vi "Agitator Settings Dialog.vi"(8 "error in (no error)":errorcluster, 10 "Message Queues":T7, 11 "Agitator Module State Cluster In":T1={"State"=enum."Idle", "Start Time"=timestamp(0 s since 1904-01-01), "Current Time"=timestamp(0 s since 1904-01-01), "Agitator Module Config"={"GUID"="", "Drop Coords"={"Horizontal"=0, "Vertical"=0}, "Process Name"="", "User name"="", "Queue Name"="", "Settings"={"Cycle Period"=500.0, "Agitator Type"="", "Setpoint (µm)"=0.0, "IKA EUROSTAR Settings"={"VISA resource name"="", "Simulated?"=FALSE}}, "Load Count"=0}, "Output Error"=FALSE, "Log Started"=FALSE, "First Iteration"=FALSE, "Data"={"Agitator rpm Value"=0.0}, "Agitator On?"=enum."Off"}) -> (0 "error out":errorcluster, 1 "Cancelled?":bool=TRUE, 2 "UI Refresh Needed?":bool, 3 "Agitator Module State Cluster Out":T1={"State"=enum."Idle", "Start Time"=timestamp(0 s since 1904-01-01), "Current Time"=timestamp(0 s since 1904-01-01), "Agitator Module Config"={"GUID"="", "Drop Coords"={"Horizontal"=0, "Vertical"=0}, "Process Name"="", "User name"="", "Queue Name"="", "Settings"={"Cycle Period"=500.0, "Agitator Type"="", "Setpoint (µm)"=0.0, "IKA EUROSTAR Settings"={"VISA resource name"="", "Simulated?"=FALSE}}, "Load Count"=0}, "Output Error"=FALSE, "Log Started"=FALSE, "First Iteration"=FALSE, "Data"={"Agitator rpm Value"=0.0}, "Agitator On?"=enum."Off"})   [LabVIEW 2018, in "Agitator Module.lvlib"]
doc: "Dialog for selecting user specified settings."
uses:
  Agitator Module.lvlib
  Feed Module/Controls/Agitator Module Settings Cluster and Start Stop.ctl
  Feed Module/Controls/Agitator Module Settings Cluster.ctl
  IKA EUROSTAR/IKA EUROSTAR Settings.ctl
  Agitator Message Queues.ctl
  support/Message Queue/Message Cluster.ctl
  Feed Module/Controls/Agitator Module State Cluster.ctl
  Pump Module Folder/Measure Instrument/State Enum.ctl
  Feed Module/Controls/Agitator Module Config Cluster.ctl
  <vilib>/Utility/miscctls.llb/LVPoint32TypeDef.ctl
  support/Message Queue/Enqueue Message (Single).vi
  <vilib>/Utility/xml.llb/Write to XML File(string).vi
  Settings/Settings.lvlib
  Measure Instrument/Agitator Module Engine.lvlib
  support/Support Library.lvlib
  support/Message Queue/Message Queue.lvlib
  Pump Module Folder/Measure Instrument/Pump Module Engine.lvlib
  IKA EUROSTAR/IKA EUROSTAR.lvlib
panel:
  in  "Configuration + Buttons":T8={"Configuration"={"Cycle Period"=500.0, "Agitator Type"="", "Setpoint (µm)"=0.0, "IKA EUROSTAR Settings"={"VISA resource name"="", "Simulated?"=FALSE}}, "Stop"=FALSE, "Start"=FALSE}
  in  "Module Name":string
  in  "Cancel Button":bool
  in  "OK Button":bool
  # "Non visible portion of dialog (needed for connector pane)."
  # "Agitator Settings"
  # "Agitator Settings"
  # "Agitator Settings"
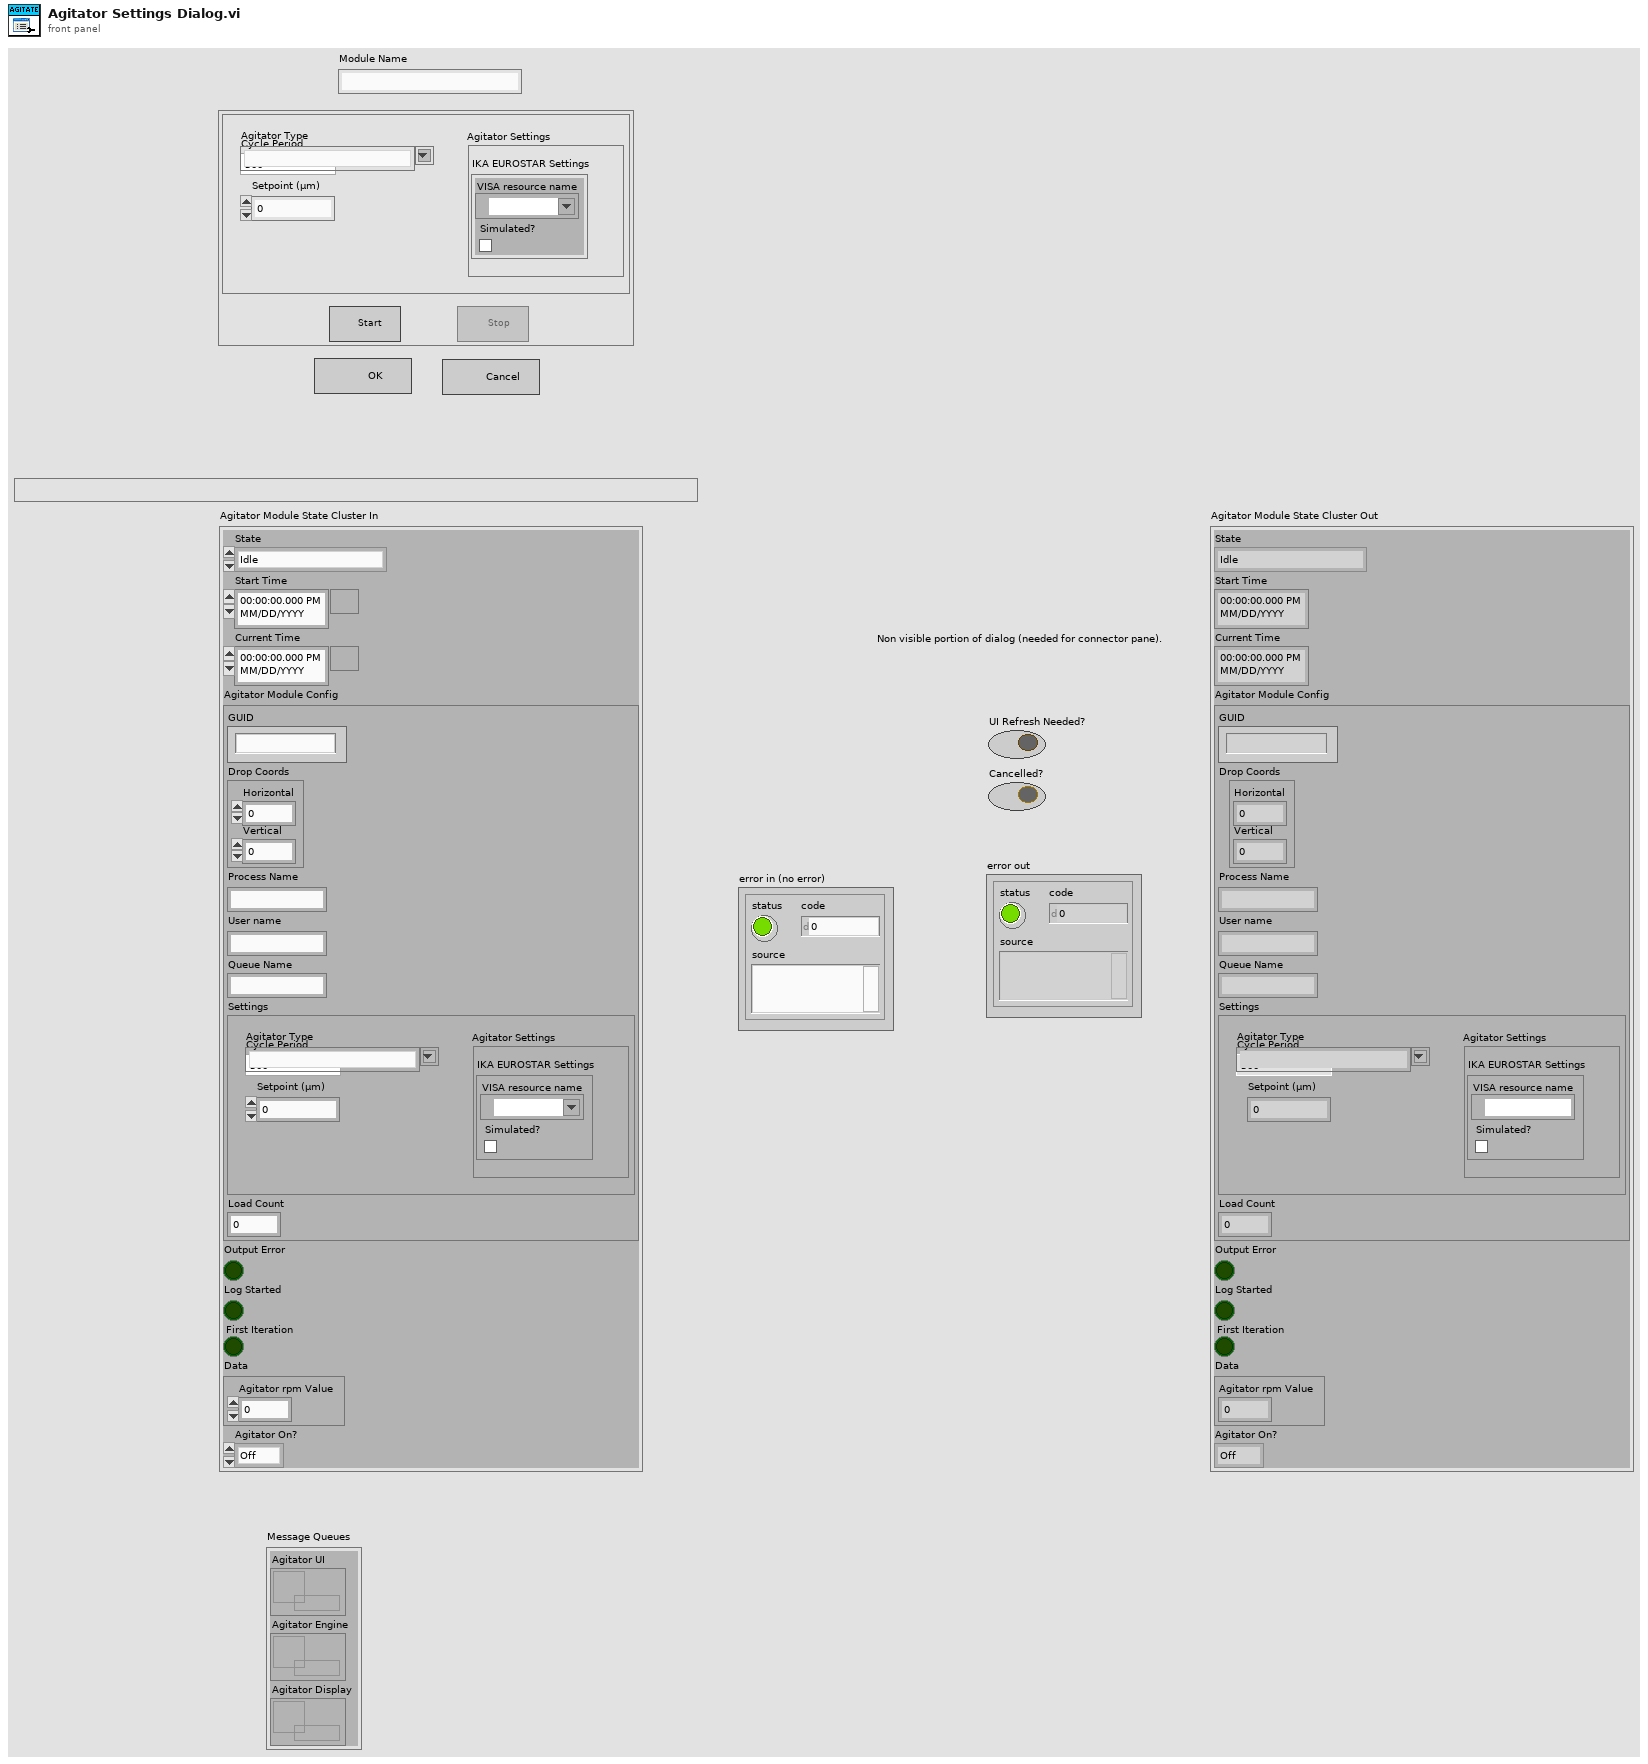
[diagram p1: front panel]
types:
  T1 = typedef "Agitator Module.lvlib/Agitator Module State Cluster.ctl" = cluster{"State":T2, "Start Time":timestamp, "Current Time":timestamp, "Agitator Module Config":T3, "Output Error":bool, "Log Started":bool, "First Iteration":bool, "Data":cluster{"Agitator rpm Value":dbl}, "Agitator On?":enum16{"Off", "On", "Not Initialized", "Over Cutoff"}}
  T2 = typedef "Pump Module.lvlib/Pump Module Engine.lvlib/State Enum.ctl" = enum16{"Measuring", "Idle", "Paused"}
  T3 = typedef "Agitator Module.lvlib/Agitator Module Config Cluster.ctl" = cluster{"GUID":string, "Drop Coords":T4, "Process Name":string, "User name":string, "Queue Name":string, "Settings":T5, "Load Count":i32}
  T4 = typedef "LVPoint32TypeDef.ctl" = cluster{"Horizontal":i32, "Vertical":i32}
  T5 = typedef "Agitator Module.lvlib/Agitator Module Settings Cluster.ctl" = cluster{"Cycle Period":dbl, "Agitator Type":string, "Setpoint (µm)":dbl, "IKA EUROSTAR Settings":T6}
  T6 = typedef "IKA EUROSTAR.lvlib/IKA EUROSTAR Settings.ctl" = cluster{"VISA resource name":refnum<visa-resource-name>, "Simulated?":bool}
  T7 = typedef "Agitator Module.lvlib/Agitator Message Queues.ctl" = cluster{"Agitator UI":refnum<queue>, "Agitator Engine":refnum<queue>, "Agitator Display":refnum<queue>}
  T8 = typedef "Agitator Module.lvlib/Agitator Module Settings Cluster and Start Stop.ctl" = cluster{"Configuration":T5, "Stop":bool, "Start":bool}
  T9 = enum8{"Enabled", "Disabled", "Disabled and Grayed Out"}
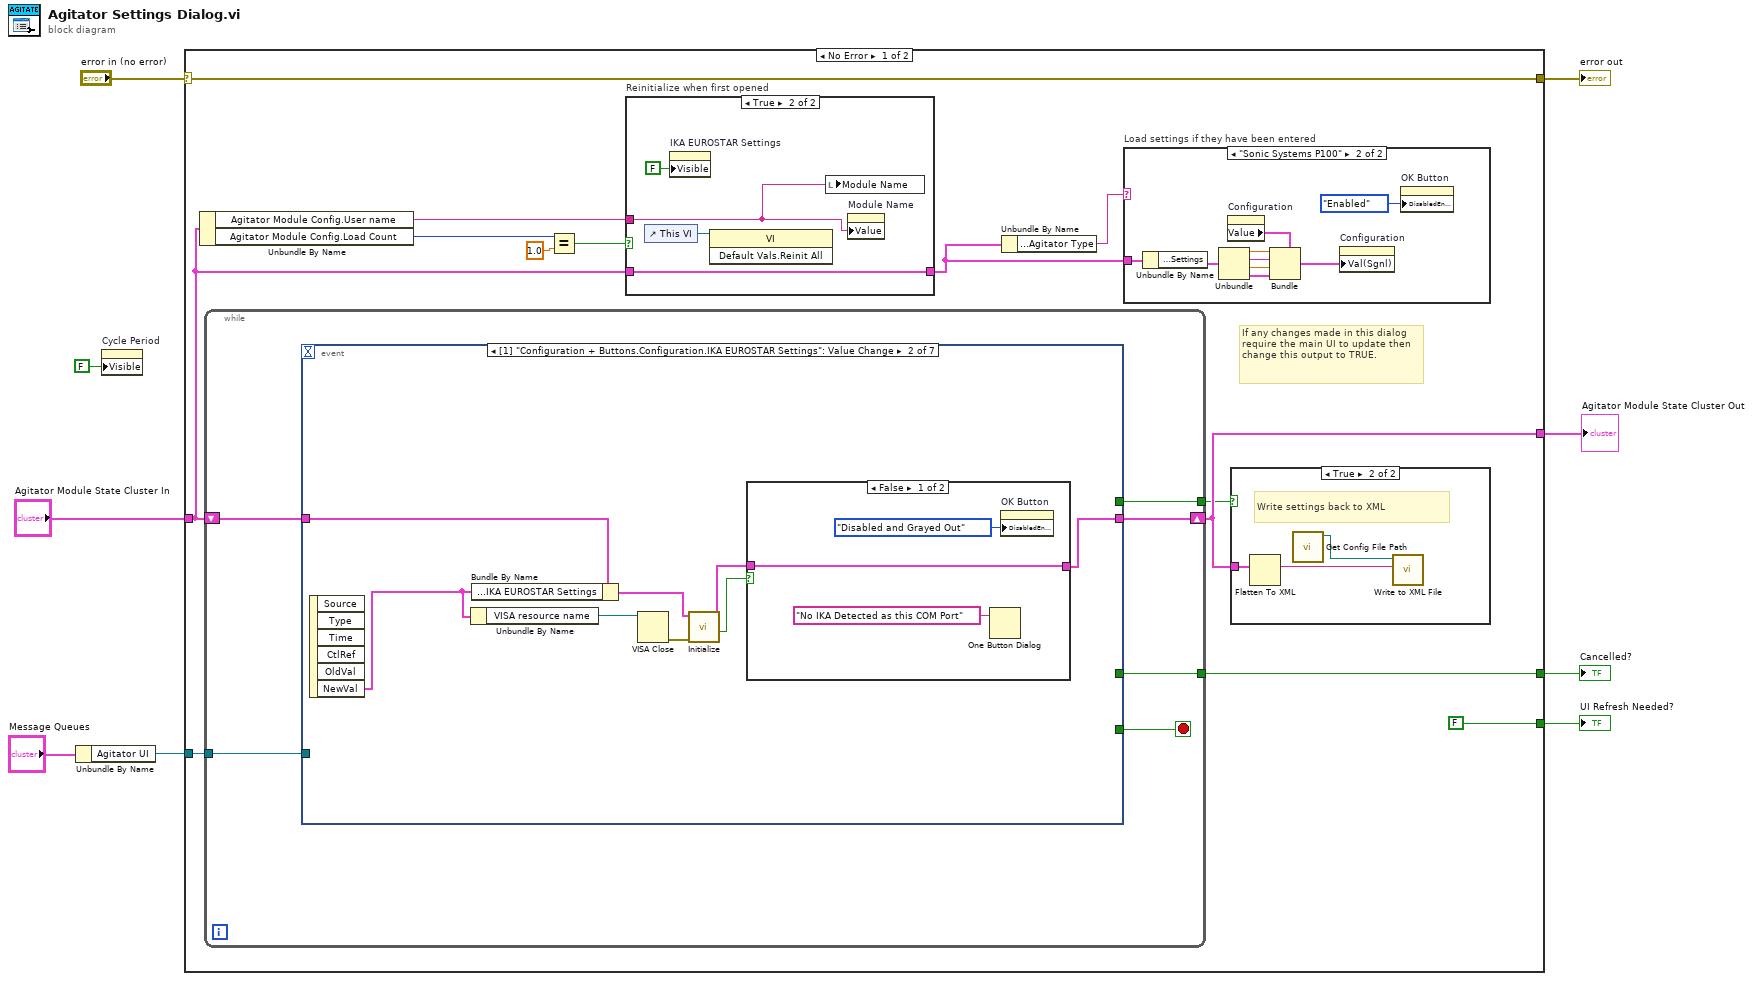
[diagram p0: block diagram]
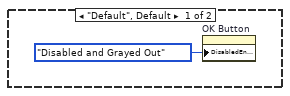
[diagram p2: hidden frame]
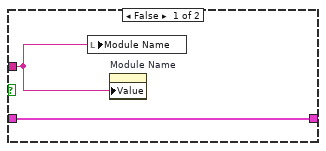
[diagram p3: hidden frame]
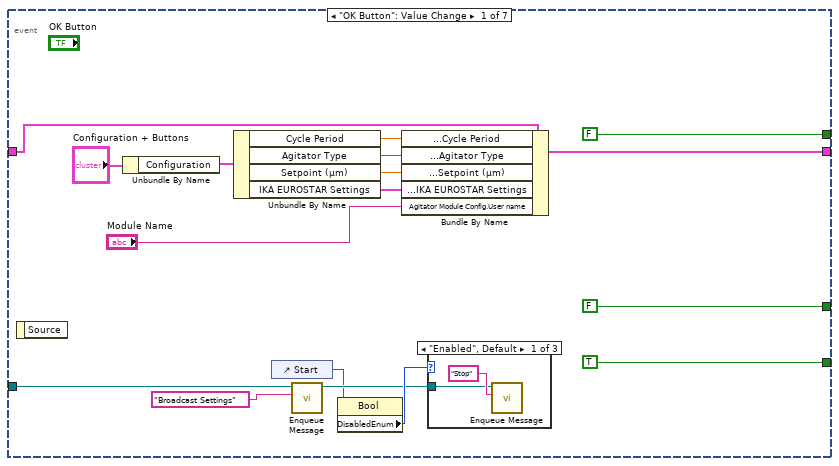
[diagram p4: hidden frame]
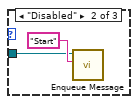
[diagram p5: hidden frame]
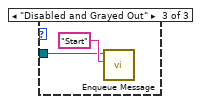
[diagram p6: hidden frame]
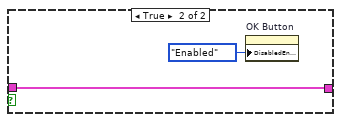
[diagram p7: hidden frame]
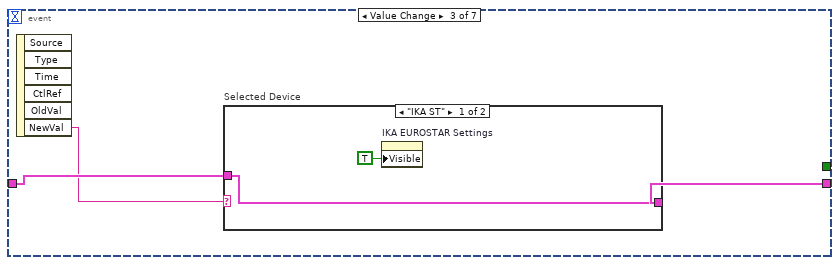
[diagram p8: hidden frame]
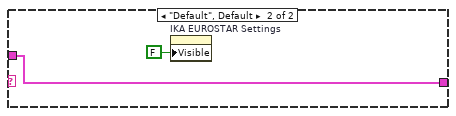
[diagram p9: hidden frame]
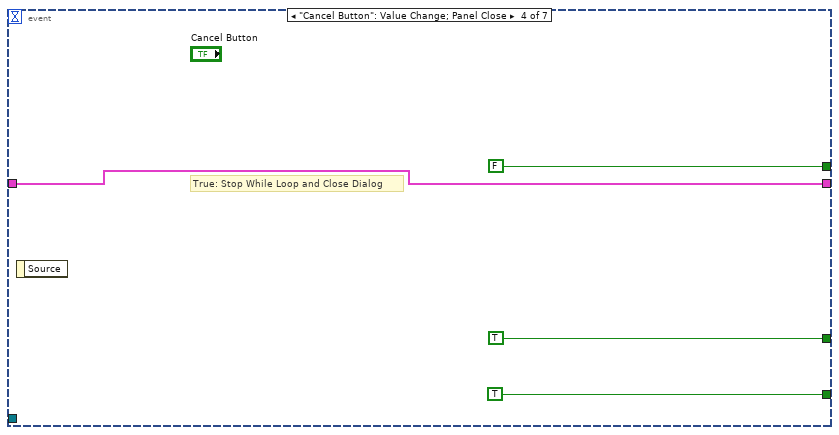
[diagram p10: hidden frame]
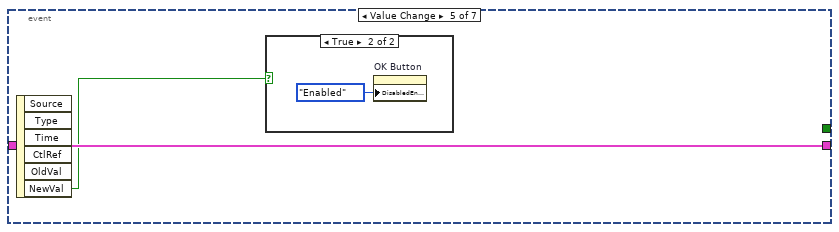
[diagram p11: hidden frame]
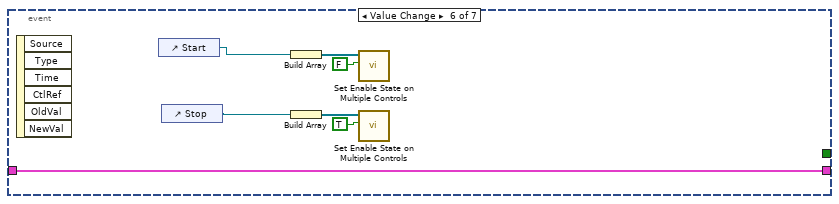
[diagram p13: hidden frame]
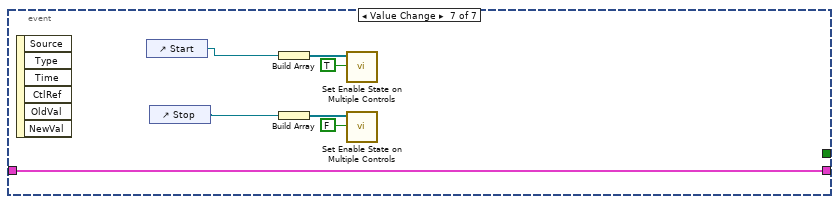
[diagram p14: hidden frame]
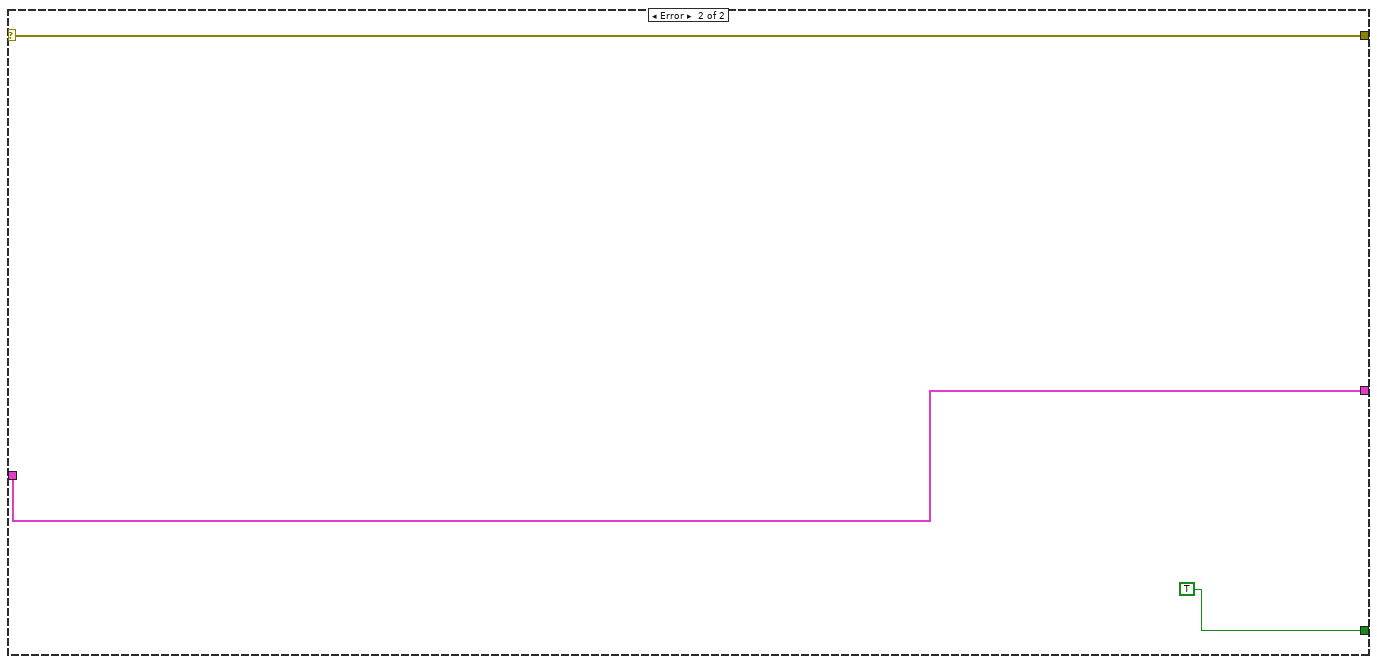
[diagram p16: hidden frame]
diagram:
  n1 = Unbundle By Name("Message Queues") -> ("Agitator UI"=w3:refnum<queue>)
  n2 = property on="Cycle Period" class="DigNum (strict)"("Visible"=FALSE) -> ()  [unwired: 2 in, 2 out]
  n3 = case shown="No Error" "error in (no error)" {
    selector: "error in (no error)" -> [w22 w114]
    tunnel: [w22 w114] -> w9
    tunnel: "Agitator Module State Cluster In" -> [w12 w113]
    tunnel: [w20 w113] -> w1
    tunnel: [FALSE ("UI Refresh Needed?") _] -> w8
    tunnel: [w16 TRUE ("UI Refresh Needed?")] -> w7
    tunnel: w3 -> [w10 _]
    frame No Error {
      # "If any changes made in this dialog require the main UI to update then change this output to TRUE."
      n4 = Unbundle By Name(w12) -> ("Agitator Module Config.User name"=w11:string, "Agitator Module Config.Load Count"=w19:i32)
      n5 = while {
        tunnel: [w44] -> w17
        tunnel: [w41] -> w16
        shift-right: [w43] -> w20
        shift-left: w12 -> [w40]
        tunnel: w10 -> [w39]
        stop <- w42 stop-if-true
        n6 = event shown="[1] \"Configuration + Buttons.Configuration.IKA EUROSTAR Settings\": Value Change" {
          selector: _ -> [_ _ _ _ _ _ _]
          dyn-events: _ -> [_ _ _ _ _ _ _]
          timeout: _ -> [_ _ _ _ _ _ _]
          tunnel: [w59 w75 w81 w91 w93 w101 w108] -> w43
          tunnel: w40 -> [w56 w73 w83 w91 w93 w101 w108]
          tunnel: [FALSE ("UI Refresh Needed?") _ _ FALSE ("UI Refresh Needed?") _ _ _] -> w44
          tunnel: [TRUE _ _ TRUE _ _ _] -> w42
          tunnel: [FALSE ("UI Refresh Needed?") _ _ TRUE ("UI Refresh Needed?") _ _ _] -> w41
          tunnel: w39 -> [w47 _ _ _ _ _ _]
          event "OK Button": Value Change {
            n7 = event-data() -> ()  [unwired: 1 in, 1 out]
            n8 = Unbundle By Name("Configuration + Buttons") -> ("Configuration"=w53:T5)
            n9 = Unbundle By Name(w53) -> ("Cycle Period"=w57:dbl, "Agitator Type"=w55:string, "Setpoint (µm)"=w52:dbl, "IKA EUROSTAR Settings"=w46:T6)
            n10 = control-ref of="Start"() -> (w48:refnum<vi>)
            n11 = call-poly "Enqueue Message.vi"("Message"="Broadcast Settings", "Message Queue"=w47) -> ("dup Message Queue"=w49:refnum<queue>)  [unwired: 8 in, 1 out]
            n12 = property class="Bool"(reference=w48) -> ("DisabledEnum"=w51:T9)  [unwired: 1 in, 2 out]
            n13 = Bundle By Name(cluster=w56, "Agitator Module Config.Settings.Cycle Period"=w57, "Agitator Module Config.Settings.Agitator Type"=w55, "Agitator Module Config.Settings.Setpoint (µm)"=w52, "Agitator Module Config.Settings.IKA EUROSTAR Settings"=w46, "Agitator Module Config.User name"="Module Name") -> (w59:T1)
            n14 = case shown="\"Enabled\", Default" w51 {
              tunnel: w49 -> [w62 w64 w66]
              frame "Enabled", Default {
                n15 = call-poly "Enqueue Message.vi"("Message"="Stop", "Message Queue"=w62) -> ()  [unwired: 8 in, 2 out]
              }
              frame "Disabled" {
                n16 = call-poly "Enqueue Message.vi"("Message"="Start", "Message Queue"=w64) -> ()  [unwired: 8 in, 2 out]
              }
              frame "Disabled and Grayed Out" {
                n17 = call-poly "Enqueue Message.vi"("Message"="Start", "Message Queue"=w66) -> ()  [unwired: 8 in, 2 out]
              }
            }
          }
          event Value Change {
            n18 = event-data() -> ("NewVal"=w69:T6)  [unwired: 1 in, 5 out]
            n19 = Unbundle By Name(w69) -> ("VISA resource name"=w68:refnum<visa-resource-name>)
            n20 = Bundle By Name(cluster=w73, "Agitator Module Config.Settings.IKA EUROSTAR Settings"=w69) -> (w72:T1)
            n21 = VISA Close(VISA resource name=w68) -> (error out=w74:errorcluster)  [unwired: 1 in]
            n22 = call "Initialize.vi"("error in (no error)"=w74, "Agitator Module State Cluster"=w72) -> ("Initialized"=w70:bool, "Agitator Module State Cluster"=w71:T1)  [unwired: 7 in, 1 out]
            n23 = case shown="False" w70 {
              tunnel: [w77 w79] -> w75
              tunnel: w71 -> [w77 w79]
              frame False {
                n24 = One Button Dialog(message="No IKA Detected as this COM Port") -> ()  [unwired: 1 in, 1 out]
                n25 = property on="OK Button" class="Bool"("DisabledEnum"=T9."Disabled and Grayed Out" ("Disabled")) -> ()  [unwired: 2 in, 2 out]
              }
              frame True {
                n26 = property on="OK Button" class="Bool"("DisabledEnum"=T9."Enabled" ("Disabled")) -> ()  [unwired: 2 in, 2 out]
              }
            }
          }
          event Value Change {
            n27 = event-data() -> ("NewVal"=w82:string)  [unwired: 1 in, 5 out]
            n28 = case "Selected Device" shown="\"IKA ST\"" w82 {
              tunnel: w83 -> [w85 w87]
              tunnel: [w85 w87] -> w81
              frame "IKA ST" {
                n29 = property on="IKA EUROSTAR Settings" class="Clust (strict)"("Visible"=TRUE) -> ()  [unwired: 2 in, 2 out]
              }
              frame "Default", Default {
                n30 = property on="IKA EUROSTAR Settings" class="Clust (strict)"("Visible"=FALSE) -> ()  [unwired: 2 in, 2 out]
              }
            }
          }
          event "Cancel Button": Value Change; Panel Close {
            # "True: Stop While Loop and Close Dialog"
            n31 = event-data() -> ()  [unwired: 1 in, 1 out]
          }
          event Value Change {
            n32 = event-data() -> ("NewVal"=w92:bool)  [unwired: 1 in, 5 out]
            n33 = case shown="True" w92 {
              frame False {
              }
              frame True {
                n34 = property on="OK Button" class="Bool"("DisabledEnum"=T9."Enabled" ("Disabled")) -> ()  [unwired: 2 in, 2 out]
              }
            }
          }
          event Value Change {
            n35 = event-data() -> ()  [unwired: 1 in, 6 out]
            n36 = control-ref of="Start"() -> (w96:refnum<vi>)
            n37 = control-ref of="Stop"() -> (w95:refnum<vi>)
            n38 = Build Array(w96) -> (w98:refnum<vi>[])
            n39 = Build Array(w95) -> (w100:refnum<vi>[])
            n40 = call "Set Enable State on Multiple Controls.vi"("Enable?"=FALSE, "Controls"=w98) -> ()  [unwired: 10 in]
            n41 = call "Set Enable State on Multiple Controls.vi"("Enable?"=TRUE, "Controls"=w100) -> ()  [unwired: 10 in]
          }
          event Value Change {
            n42 = event-data() -> ()  [unwired: 1 in, 6 out]
            n43 = control-ref of="Start"() -> (w105:refnum<vi>)
            n44 = control-ref of="Stop"() -> (w104:refnum<vi>)
            n45 = Build Array(w105) -> (w106:refnum<vi>[])
            n46 = Build Array(w104) -> (w107:refnum<vi>[])
            n47 = call "Set Enable State on Multiple Controls.vi"("Enable?"=TRUE, "Controls"=w106) -> ()  [unwired: 10 in]
            n48 = call "Set Enable State on Multiple Controls.vi"("Enable?"=FALSE, "Controls"=w107) -> ()  [unwired: 10 in]
          }
        }
      }
      n49 = Equal?(x=w19, y=1.0) -> (x = y?=w15:bool)
      n50 = case "Reinitialize when first opened" shown="True" w15 {
        tunnel: w12 -> [w34 w37]
        tunnel: [w34 w37] -> w13
        tunnel: w11 -> [w33 w36]
        frame False {
          n51 = local write "Module Name"(w33) -> ()
          n52 = property on="Module Name" class="Str"("Value"=w33) -> ()  [unwired: 2 in, 2 out]
        }
        frame True {
          n53 = control-ref of="This VI"() -> (w38:refnum<vi>)
          n54 = property on="IKA EUROSTAR Settings" class="Clust (strict)"("Visible"=FALSE) -> ()  [unwired: 2 in, 2 out]
          n55 = invoke class="VI" method="Default Vals.Reinit All"(reference=w38) -> ()  [unwired: 2 in, 3 out]
          n56 = local write "Module Name"(w36) -> ()
          n57 = property on="Module Name" class="Str"("Value"=w36) -> ()  [unwired: 2 in, 2 out]
        }
      }
      n58 = Unbundle By Name(w13) -> ("Agitator Module Config.Settings.Agitator Type"=w14:string)
      n59 = case "Load settings if they have been entered" shown="\"Sonic Systems P100\"" w14 {
        tunnel: w13 -> [_ w28]
        frame "Default", Default {
          n60 = property on="OK Button" class="Bool"("DisabledEnum"=T9."Disabled and Grayed Out" ("Disabled")) -> ()  [unwired: 2 in, 2 out]
        }
        frame "Sonic Systems P100" {
          n61 = Unbundle By Name(w28) -> ("Agitator Module Config.Settings"=w30:T5)
          n62 = Unbundle(w30) -> ("Cycle Period"=w31:dbl, "Agitator Type"=w32:string, "Setpoint (µm)"=w29:dbl, "IKA EUROSTAR Settings"=w24:T6)
          n63 = property on="Configuration" class="Clust (strict)"() -> ("Value"=w26:T5)  [unwired: 2 in, 2 out]
          n64 = Bundle(cluster=w26, "Cycle Period"=w31, "Agitator Type"=w32, "Setpoint (µm)"=w29, "IKA EUROSTAR Settings"=w24) -> (w25:T5)
          n65 = property on="Configuration" class="Clust (strict)"("Val(Sgnl)"=w25) -> ()  [unwired: 2 in, 2 out]
          n66 = property on="OK Button" class="Bool"("DisabledEnum"=T9."Enabled" ("Disabled")) -> ()  [unwired: 2 in, 2 out]
        }
      }
      n67 = case shown="True" w17 {
        tunnel: w20 -> [_ w110]
        frame False {
        }
        frame True {
          # "Write settings back to XML"
          n68 = Flatten To XML(anything=w110) -> (xml string=w109:string)
          n69 = call "Get Config File Path.vi"() -> ("XML File Path"=w111:path)  [unwired: 10 in, 1 out]
          n70 = call-poly <vilib>:"Write to XML File.vi"("XML Input"=w109, "XML File Path"=w111) -> ()  [unwired: 7 in, 3 out]
        }
      }
    }
    frame Error {
    }
  }
  "UI Refresh Needed?" <- w8
  "error out" <- w9
  "Cancelled?" <- w7
  "Agitator Module State Cluster Out" <- w1
